vi "错误说明.vi"(11 "code":i32) -> ()   [LabVIEW 2014]
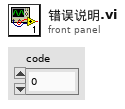
[diagram p1: front panel]
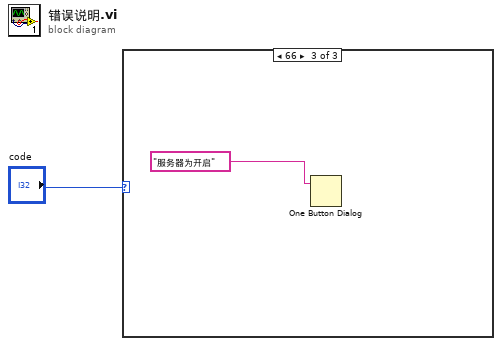
[diagram p0: block diagram]
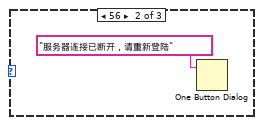
[diagram p3: hidden frame]
diagram:
  n1 = case shown="66" "code" {
    frame 0, Default {
    }
    frame 56 {
      n2 = One Button Dialog(message="服务器连接已断开，请重新登陆") -> ()  [unwired: 1 in, 1 out]
    }
    frame 66 {
      n3 = One Button Dialog(message="服务器为开启") -> ()  [unwired: 1 in, 1 out]
    }
  }
